vi "Measure.vi"(8 "error in (no error)":errorcluster, 9 "measurement configuration":variant, 10 "measure call context in":refnum<class "Measure Call Context.lvclass">, 11 "measurement plugin service in":refnum<class "Measurement Plugin Service.lvclass">) -> (0 "error out":errorcluster, 1 "measurement results":variant, 2 "measure call context out":refnum<class "Measure Call Context.lvclass">, 3 "measurement plugin service out":refnum<class "Measurement Plugin Service.lvclass">)   [LabVIEW 2021, in "NI Measurement Plug-In SDK.lvlib" / "Measurement Plugin Service.lvclass"]
doc: "Executes the measurement."
uses:
  Measurement Plugin Service.lvclass
  Measure Call Context/Measure Call Context.lvclass
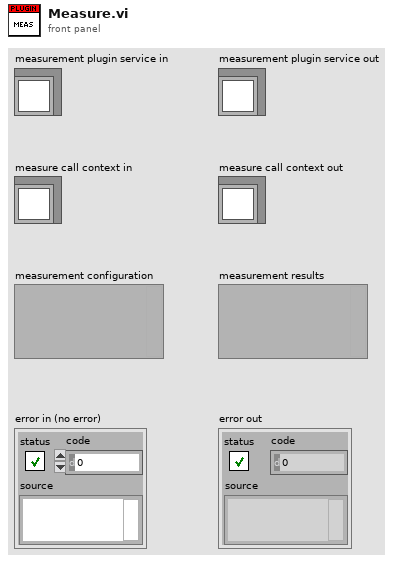
[diagram p1: front panel]
types:
  T1 = typedef "NI Measurement Plug-In SDK.lvlib/Measurement Plugin Service.lvclass/Plugin Paths.ctl" = cluster{"get service descriptor VI path":path, "get type specializations VI path":path, "get UI details VI path":path, "measurement logic VI path":path, "measurement configuration ctl path":path, "measurement results ctl path":path}
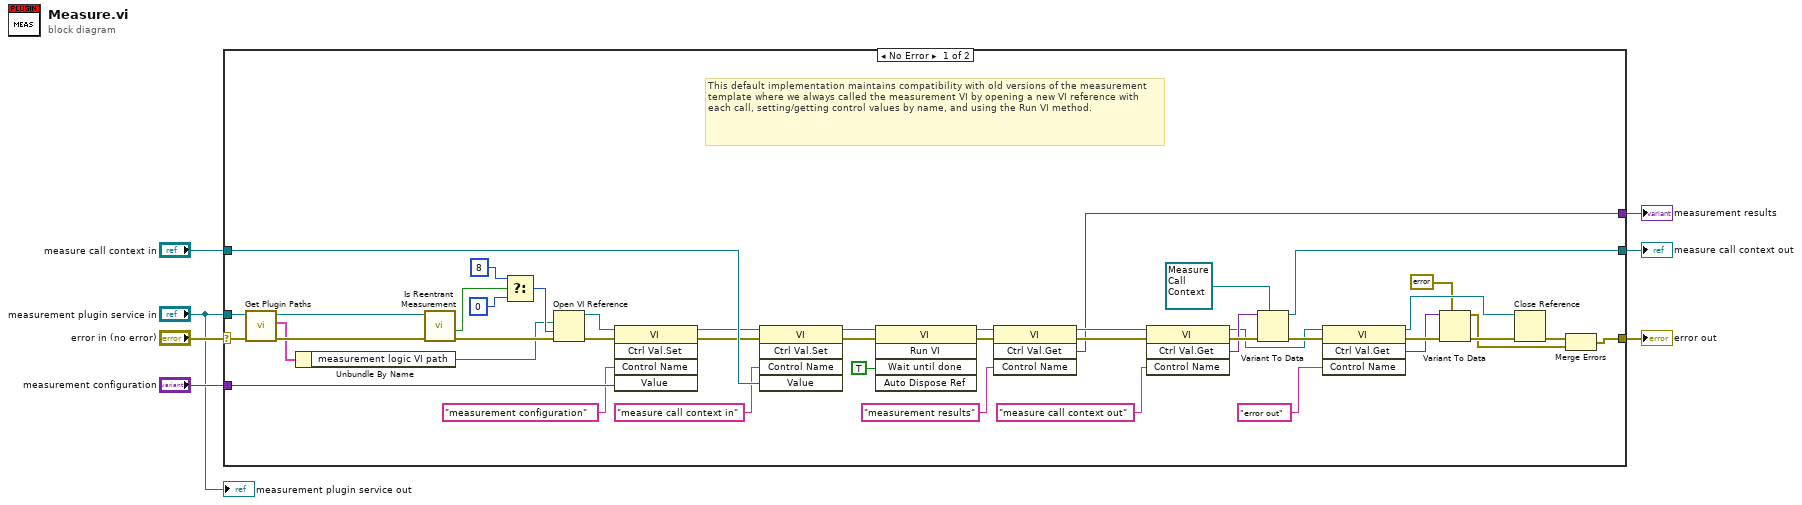
[diagram p0: block diagram]
diagram:
  n1 = case shown="No Error" "error in (no error)" {
    selector: "error in (no error)" -> [w15 w52]
    tunnel: [w51 w53] -> w4
    tunnel: "measure call context in" -> [w43 w53]
    tunnel: [w42 _] -> w6
    tunnel: "measurement configuration" -> [w41 _]
    tunnel: [w16 w52] -> w2
    tunnel: "measurement plugin service in" -> [w14 _]
    frame No Error {
      # "This default implementation maintains compatibility with old versions of the measurement template where we always called the measurement VI by opening a new VI reference with each call, setting/getting control values by name, and using the Run VI method."
      n2 = call-dynamic "Get Plugin Paths.vi"("error in"=w15, "measurement plugin service in"=w14) -> ("error out"=w13:errorcluster, "plugin paths"=w9:T1, "measurement plugin service out"=w12:refnum<class "Measurement Plugin Service.lvclass">)  [unwired: 7 in]
      n3 = Unbundle By Name(w9) -> ("measurement logic VI path"=w8:path)
      n4 = call "Is Reentrant Measurement.vi"("error in (no error)"=w13, "measurement plugin service in"=w12) -> ("error out"=w10:errorcluster, "is reentrant"=w11:bool)  [unwired: 7 in, 1 out]
      n5 = Select(t=8 ("options"), s=w11, f=0 ("options")) -> (s? t:f=w19:i32)
      n6 = Open VI Reference(vi path=w8, options=w19, error in (no error)=w10) -> (vi reference=w22:refnum<vi>, error out=w23:errorcluster)  [unwired: 3 in]
      n7 = invoke class="VI" method="Ctrl Val.Set"(reference=w22, error in=w23, "Control Name"="measurement configuration", "Value"=w41) -> (reference out=w28:refnum<vi>, error out=w29:errorcluster)  [unwired: 1 in, 3 out]
      n8 = invoke class="VI" method="Ctrl Val.Set"(reference=w28, error in=w29, "Control Name"="measure call context in", "Value"=w43) -> (reference out=w32:refnum<vi>, error out=w31:errorcluster)  [unwired: 1 in, 3 out]
      n9 = invoke class="VI" method="Run VI"(reference=w32, error in=w31, "Wait until done"=TRUE ("Wait Until Done")) -> (reference out=w34:refnum<vi>, error out=w35:errorcluster)  [unwired: 2 in, 3 out]
      n10 = invoke class="VI" method="Ctrl Val.Get"(reference=w34, error in=w35, "Control Name"="measurement results") -> (reference out=w44:refnum<vi>, error out=w46:errorcluster, "Get Control Value Variant"=w42:variant)  [unwired: 1 in, 1 out]
      n11 = invoke class="VI" method="Ctrl Val.Get"(reference=w44, error in=w46, "Control Name"="measure call context out") -> (reference out=w45:refnum<vi>, error out=w49:errorcluster, "Get Control Value Variant"=w48:variant)  [unwired: 1 in, 1 out]
      n12 = Variant To Data(error in=w49, type=refnum<class "Measure Call Context.lvclass"> refnum ("MeasurementContext in"), Variant=w48) -> (data=w51:refnum<class "Measure Call Context.lvclass">, error out=w50:errorcluster)
      n13 = invoke class="VI" method="Ctrl Val.Get"(reference=w45, error in=w50, "Control Name"="error out") -> (reference out=w38:refnum<vi>, error out=w39:errorcluster, "Get Control Value Variant"=w37:variant)  [unwired: 1 in, 1 out]
      n14 = Variant To Data(error in=w39, type=errorcluster {"status"=FALSE, "code"=0, "source"=""} ("error out"), Variant=w37) -> (data=w17:errorcluster, error out=w40:errorcluster)
      n15 = Close Reference(reference=w38, error in (no error)=w40) -> (error out=w18:errorcluster)
      n16 = Merge Errors(w18, w17) -> (w16:errorcluster)
    }
    frame Error {
    }
  }
  "error out" <- w2
  "measure call context out" <- w4
  "measurement results" <- w6
  "measurement plugin service out" <- "measurement plugin service in"
